vi "memory_load_B_2.vi"() -> (0 "Init Data Out":fxp<+/-,32,16>)   [LabVIEW 2020]
panel:
  # "For Initialization VI requirements and help, please read directions located on Block Diagram."
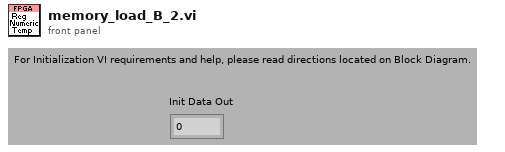
[diagram p1: front panel]
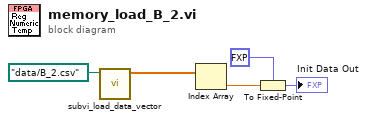
[diagram p0: block diagram]
diagram:
  n1 = call "subvi_load_data_vector.vi"("default name"=path "data/B_2.csv") -> ("array type (2D Dbl) out"=w4:dbl[])  [unwired: 10 in]
  n2 = Index Array(array=w4) -> (element=w2:dbl)  [unwired: 1 in]
  n3 = To Fixed-Point(fixed-point type=fxp<+/-,32,16> 0.0 ("fixed-point"), number=w2) -> (fixed-point=→"Init Data Out":fxp<+/-,32,16>)
